vi "DataAcqRecordPathGlobal.vi"() -> ()   [LabVIEW 2013, in "main.lvlib"]
uses:
  main.lvlib
panel:
  in  "CalibrationOffset":dbl
  in  "PressureCalibrationFactor":dbl
  in  "DataAcqState":string
  in  "DataAcqRecordPath":path
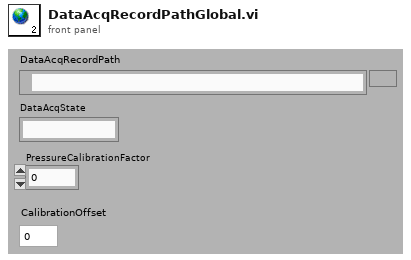
[diagram p1: front panel]
diagram:
